vi "ev i change.vi"(8 "error in (no error)":errorcluster, 11 "IDE simple in":refnum<class "LF2R IDE.lvclass">) -> (0 "error out":errorcluster, 3 "IDE simple out":refnum<class "LF2R IDE.lvclass">)   [LabVIEW 2018, in "LF2R IDE.lvlib" / "LF2R IDE.lvclass"]
uses:
  LF2R IDE.lvclass
  LF2R IDE.lvclass/LF2R IDE.ctl
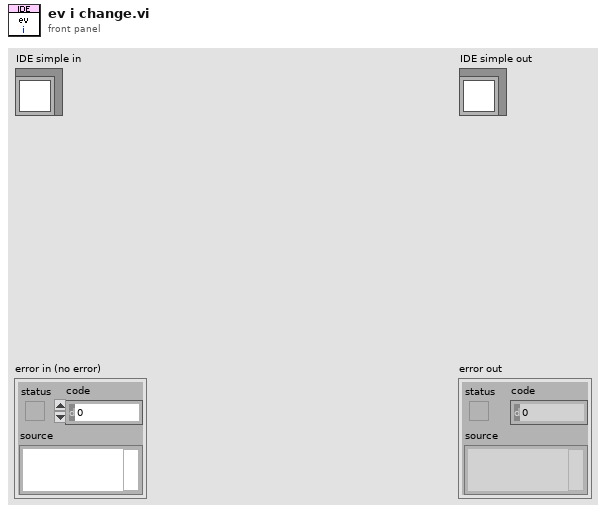
[diagram p1: front panel]
types:
  T1 = typedef "Frame Analizer.lvclass/frame i data.ctl" = cluster{"kind":string, "x":string, "y":string, "w":string, "h":string, "dvx":string, "dvy":string, "dvz":string, "fall":string, "arest":string, "vrest":string, "bdefend":string, "injury":string, "zwidth":string, "effect":string, "catchingact":string, "caughtact":string}
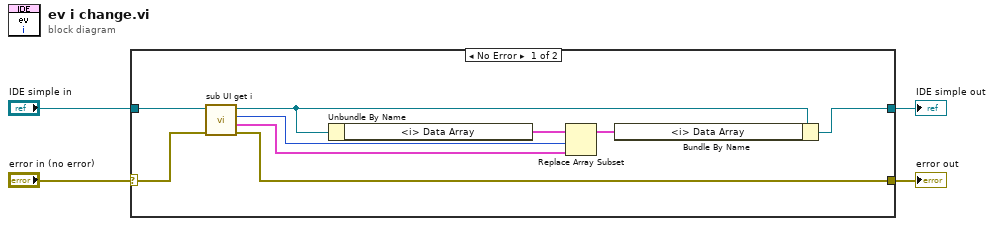
[diagram p0: block diagram]
diagram:
  n1 = case shown="No Error" "error in (no error)" {
    selector: "error in (no error)" -> [w12 w15]
    tunnel: [w11 w15] -> w3
    tunnel: [w10 w14] -> w1
    tunnel: "IDE simple in" -> [w13 w14]
    frame No Error {
      n2 = call "sub UI get i.vi"("error in (no error)"=w12, "IDE simple in"=w13) -> ("error out"=w11:errorcluster, "<i> data"=w5:T1, "index"=w6:u32, "IDE simple out"=w9:refnum<class "LF2R IDE.lvclass">)  [unwired: 6 in]
      n3 = Unbundle By Name(w9) -> ("<i> Data Array"=w8:T1[])
      n4 = Replace Array Subset(array=w8, new element=w5, index=w6) -> (w7:T1[])
      n5 = Bundle By Name(cluster=w9, "<i> Data Array"=w7) -> (w10:refnum<class "LF2R IDE.lvclass">)
    }
    frame Error {
    }
  }
  "error out" <- w3
  "IDE simple out" <- w1
